vi "last_modified.get.vi"(11 "comic_class in":refnum<class "comic_class.lvclass">) -> (2 "last modified":timestamp, 3 "comic_class out":refnum<class "comic_class.lvclass">)   [LabVIEW 2024, in "comic_class.lvclass"]
uses:
  comic_class.lvclass
  comic_class.lvclass/comic_class.ctl
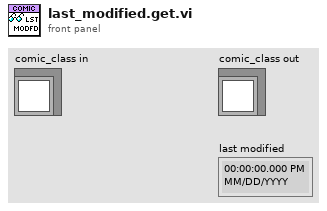
[diagram p1: front panel]
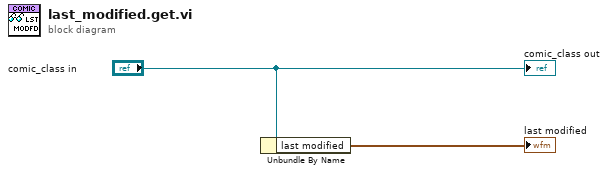
[diagram p0: block diagram]
diagram:
  n1 = Unbundle By Name("comic_class in") -> ("last modified"=→"last modified":timestamp)
  "comic_class out" <- "comic_class in"
